vi "QCA Read Setup File.vi"(1 "error in (no error)":errorcluster, 2 "setup file":path) -> (0 "error out":errorcluster)   [LabVIEW 2010]
uses:
  QCA Global.vi
  <vilib>/Utility/config.llb/Read Key (Path).vi
  <vilib>/Utility/config.llb/NI_LVConfig.lvlib
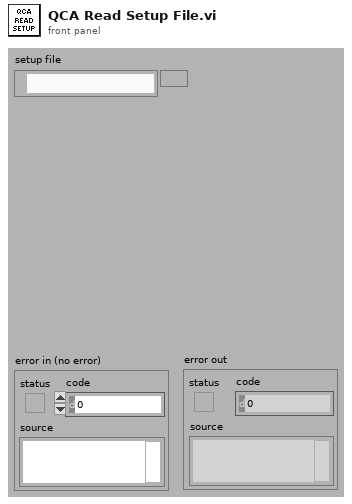
[diagram p1: front panel]
types:
  T1 = typedef "NI_LVConfig.lvlib/Config Data RefNum.ctl" = refnum<k1>
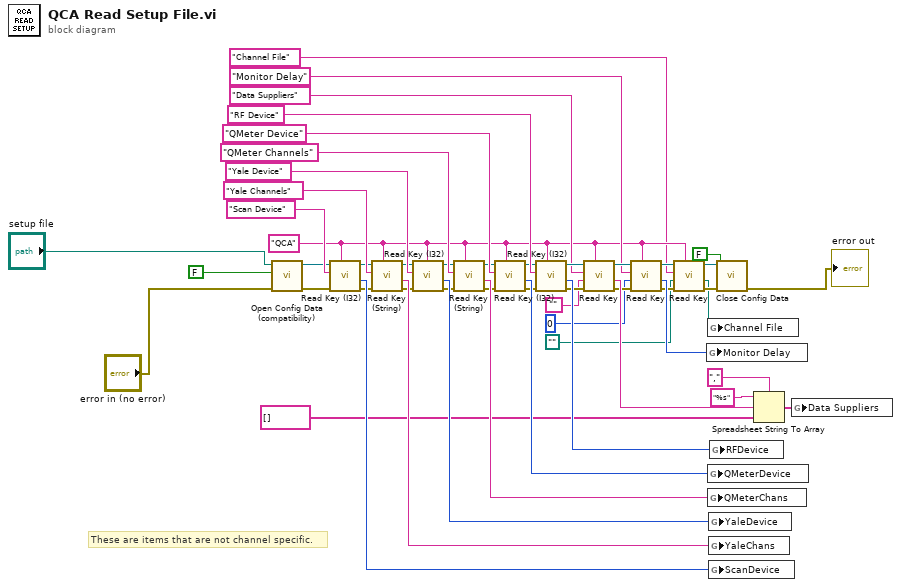
[diagram p0: block diagram]
diagram:
  w8 = "QCA" ("section")
  # "These are items that are not channel specific."
  n1 = call <vilib>:"Open Config Data (compatibility).vi"("error in (no error)"="error in (no error)", "create file if necessary (T)"=FALSE ("create file if necessary? (T)"), "configuration file path"="setup file") -> ("error out"=w49:errorcluster, "refnum"=w50:T1)  [unwired: 6 in, 1 out]
  n2 = call <vilib>:"Read Key (I32).vi"("section"=w8, "error in (no error)"=w49, "key"="Scan Device", "refnum"=w50) -> ("error out"=w36:errorcluster, "value"=w47:i32, "refnum out"=w27:T1)  [unwired: 4 in, 1 out]
  n3 = call <vilib>:"Read Key (String).vi"("section"=w8, "error in (no error)"=w36, "key"="Yale Channels", "refnum"=w27) -> ("error out"=w35:errorcluster, "value"=w46:string, "refnum out"=w28:T1)  [unwired: 4 in, 1 out]
  n4 = call <vilib>:"Read Key (I32).vi"("section"=w8, "error in (no error)"=w35, "key"="Yale Device", "refnum"=w28) -> ("error out"=w34:errorcluster, "value"=w43:i32, "refnum out"=w29:T1)  [unwired: 4 in, 1 out]
  n5 = call <vilib>:"Read Key (String).vi"("section"=w8, "error in (no error)"=w34, "key"="QMeter Channels", "refnum"=w29) -> ("error out"=w33:errorcluster, "value"=w42:string, "refnum out"=w30:T1)  [unwired: 4 in, 1 out]
  n6 = call <vilib>:"Read Key (I32).vi"("section"=w8, "error in (no error)"=w33, "key"="QMeter Device", "refnum"=w30) -> ("error out"=w32:errorcluster, "value"=w39:i32, "refnum out"=w31:T1)  [unwired: 4 in, 1 out]
  n7 = call <vilib>:"Read Key (I32).vi"("section"=w8, "error in (no error)"=w32, "key"="RF Device", "refnum"=w31) -> ("error out"=w26:errorcluster, "value"=w38:i32, "refnum out"=w25:T1)  [unwired: 4 in, 1 out]
  n8 = call-poly <vilib>:"Read Key.vi"("section"=w8, "error in (no error)"=w26, "default value"="", "key"="Data Suppliers", "refnum"=w25) -> ("error out"=w18:errorcluster, "value"=w22:string, "refnum out"=w17:T1)  [unwired: 3 in, 1 out]
  n9 = call-poly <vilib>:"Read Key.vi"("section"=w8, "error in (no error)"=w18, "default value"=0, "key"="Monitor Delay", "refnum"=w17) -> ("error out"=w12:errorcluster, "value"=w14:i32, "refnum out"=w11:T1)  [unwired: 3 in, 1 out]
  n10 = call-poly <vilib>:"Read Key.vi"("section"=w8, "error in (no error)"=w12, "default value"=path "", "key"="Channel File", "refnum"=w11) -> ("error out"=w10:errorcluster, "value"=w6:path, "refnum out"=w9:T1)  [unwired: 3 in, 1 out]
  n11 = global write "QCA Global.vi" "Monitor Delay"(w14) -> ()
  n12 = global write "QCA Global.vi" "Channel File"(w6) -> ()
  n13 = global write "QCA Global.vi" "QMeterDevice"(w39) -> ()
  n14 = global write "QCA Global.vi" "QMeterChans"(w42) -> ()
  n15 = global write "QCA Global.vi" "YaleDevice"(w43) -> ()
  n16 = global write "QCA Global.vi" "YaleChans"(w46) -> ()
  n17 = global write "QCA Global.vi" "ScanDevice"(w47) -> ()
  n18 = global write "QCA Global.vi" "RFDevice"(w38) -> ()
  n19 = call <vilib>:"Close Config Data.vi"("error in (no error)"=w10, "write file if changed (T)"=FALSE, "refnum"=w9) -> ("error out"=→"error out":errorcluster)  [unwired: 7 in, 1 out]
  n20 = Spreadsheet String To Array(delimiter (Tab)=",", format string="%s", spreadsheet string=w22, array type (2D Dbl)=string[] [] ("Array Constant")) -> (array=w19:string[])
  n21 = global write "QCA Global.vi" "Data Suppliers"(w19) -> ()
